vi "Query Multi Eval Meas Status.vi"(8 "error in (no error)":errorcluster, 10 "Instance (1)":T1=1, 11 "VISA resource name":refnum<visa-resource-name>) -> (0 "error out":errorcluster, 1 "Sync State":i32, 2 "Main State":i32, 3 "VISA resource name out":refnum<visa-resource-name>, 4 "Resources State":i32)   [LabVIEW 2015, in "Rohde&Schwarz CMXP NR FR2 Measurement.lvlib"]
doc: "Queries the main measurement state and the measurement substates. Both measurement substates are relevant for running measurements only. Use FETCh:...:STATe? to query the main measurement state only. Use INITiate..., STOP..., ABORt... to change the measurement state.\n\nAttribute:\nRSCMXPNRFR2M_ATTR_MULTI_EVAL_MEASUREMENT_MEASUREMENT_STATE\n\nRemote-control command:\nFETCh:NRMMw:MEAS<i>:MEValuation:STATe:ALL?"
uses:
  <instrlib>/Rohde&Schwarz CMXP NR FR2 Measurement/Rohde&Schwarz CMXP NR FR2 Measurement.lvlib
  <instrlib>/Rohde&Schwarz CMXP NR FR2 Measurement/Private/_Instance.ctl
  <instrlib>/Rohde&Schwarz CMXP NR FR2 Measurement/Private/rsidr_core.llb/rsidr_core.lvlib
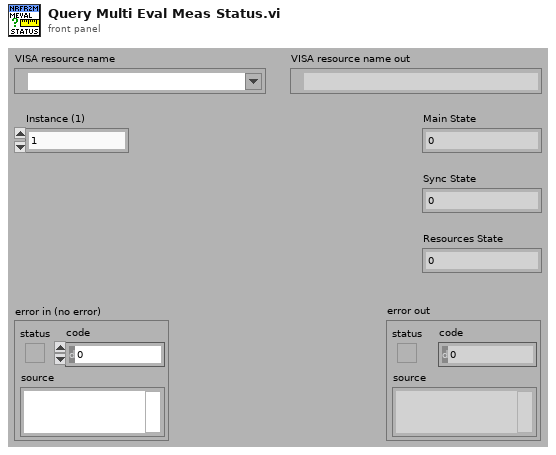
[diagram p1: front panel]
types:
  T1 = typedef "Rohde&Schwarz CMXP NR FR2 Measurement.lvlib/_Instance.ctl" = i32
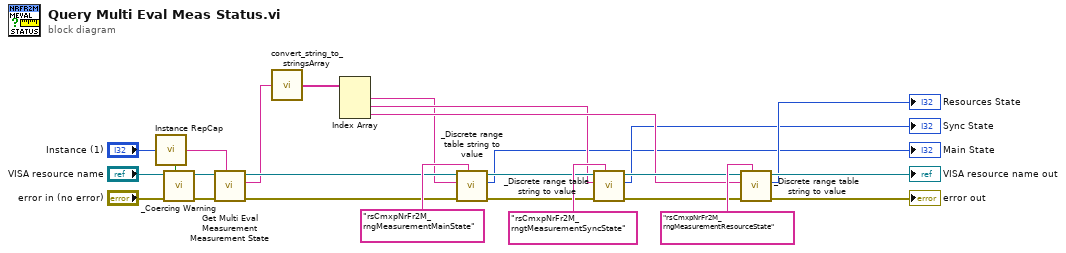
[diagram p0: block diagram]
diagram:
  n1 = call <instrlib>:"Instance RepCap.vi"("Instance In"="Instance (1)") -> ("In Range?"=w25:bool, "RepCap Identifier Out"=w21:string)  [unwired: 1 in]
  n2 = call <instrlib>:"_Coercing Warning.vi"("In Range?"=w25, "error in (no error)"="error in (no error)", "VISA resource name"="VISA resource name") -> ("error out"=w22:errorcluster, "VISA resource name out"=w23:refnum<visa-resource-name>)  [unwired: 7 in]
  n3 = call "Get Multi Eval Measurement Measurement State"("Repeated Capabilities"=w21, "error in (no error)"=w22, "instrument handle"=w23) -> ("error out"=w19:errorcluster, "Multi Eval Measurement Measurement State"=w1:string, "instrument handle out"=w18:refnum<visa-resource-name>)  [unwired: 6 in]
  n4 = call <instrlib>:"convert_string_to_stringsArray.vi"("String in"=w1) -> ("string array out"=w17:string[])  [unwired: 3 in, 1 out]
  n5 = Index Array(array=w17) -> (element #1=w8:string, element #2=w9:string, element #3=w10:string)  [unwired: 3 in]
  n6 = call <instrlib>:"_Discrete range table string to value.vi"("Discrete Range Table Identifier"="rsCmxpNrFr2M_rngMeasurementMainState", "error in (no error)"=w19, "String Value In"=w8, "VISA resource name"=w18) -> ("error out"=w15:errorcluster, "Enum Value"=→"Main State":i32, "VISA resource name out"=w11:refnum<visa-resource-name>)  [unwired: 5 in]
  n7 = call <instrlib>:"_Discrete range table string to value.vi"("Discrete Range Table Identifier"="rsCmxpNrFr2M_rngtMeasurementSyncState", "error in (no error)"=w15, "String Value In"=w9, "VISA resource name"=w11) -> ("error out"=w13:errorcluster, "Enum Value"=→"Sync State":i32, "VISA resource name out"=w12:refnum<visa-resource-name>)  [unwired: 5 in]
  n8 = call <instrlib>:"_Discrete range table string to value.vi"("Discrete Range Table Identifier"="rsCmxpNrFr2M_rngMeasurementResourceState", "error in (no error)"=w13, "String Value In"=w10, "VISA resource name"=w12) -> ("error out"=→"error out":errorcluster, "Enum Value"=→"Resources State":i32, "VISA resource name out"=→"VISA resource name out":refnum<visa-resource-name>)  [unwired: 5 in]
